vi "cwlaserOnOff.vi"(2 "error in":errorcluster, 3 "Laser On/Off":bool, 4 "cwlaser in":refnum<visa-resource-name>) -> (0 "error out":errorcluster, 1 "cwlaser out":refnum<visa-resource-name>)   [LabVIEW 2017]
panel:
  out "read buffer 3":string
  out "read buffer 2":string
  out "read buffer":string
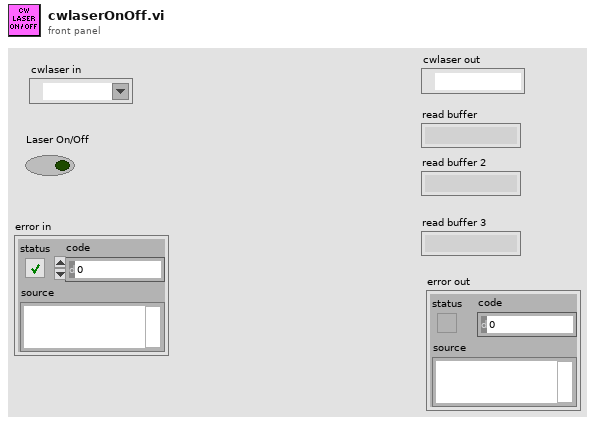
[diagram p1: front panel]
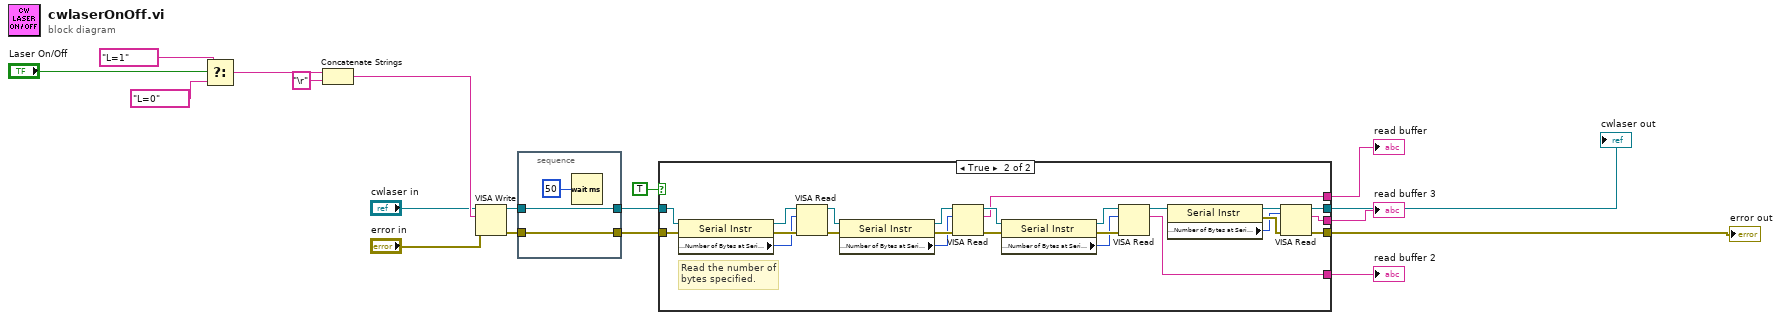
[diagram p0: block diagram]
diagram:
  n1 = Select(t="L=1" ("OutString"), s="Laser On/Off", f="L=0" ("OutString")) -> (s? t:f=w4:string)
  n2 = Concatenate Strings "Concatenate Strings"(w4, "\r") -> (w11:string)
  n3 = VISA Write(VISA resource name="cwlaser in", write buffer=w11, error in (no error)="error in") -> (VISA resource name out=w15:refnum<visa-resource-name>, error out=w14:errorcluster)  [unwired: 1 out]
  n4 = stacked-sequence {
    tunnel: w14 -> [w21]
    tunnel: [w21] -> w16
    tunnel: w15 -> [w20]
    tunnel: [w20] -> w17
    frame #0 {
      n5 = Wait (ms)(milliseconds to wait=u32 50 ("delay before read (ms)")) -> ()  [unwired: 1 out]
    }
  }
  n6 = case shown="True" TRUE ("read") {
    tunnel: w16 -> [w23 w35]
    tunnel: [w23 w25] -> w8
    tunnel: [w22 w26] -> w1
    tunnel: w17 -> [w22 w36]
    tunnel: [_ w37] -> w10
    tunnel: [_ w31] -> w13
    tunnel: [_ w24] -> w12
    frame False {
    }
    frame True {
      # "Read the number of bytes specified."
      n7 = property class="Serial Instr"(reference=w36, error in=w35) -> (reference out=w34:refnum<visa-resource-name>, error out=w33:errorcluster, "Serial Settings:Number of Bytes at Serial Port"=w32:u32)
      n8 = VISA Read(VISA resource name=w34, byte count=w32, error in (no error)=w33) -> (VISA resource name out=w41:refnum<visa-resource-name>, error out=w40:errorcluster)  [unwired: 2 out]
      n9 = property class="Serial Instr"(reference=w41, error in=w40) -> (reference out=w43:refnum<visa-resource-name>, error out=w42:errorcluster, "Serial Settings:Number of Bytes at Serial Port"=w39:u32)
      n10 = VISA Read(VISA resource name=w43, byte count=w39, error in (no error)=w42) -> (VISA resource name out=w45:refnum<visa-resource-name>, read buffer=w37:string, error out=w44:errorcluster)  [unwired: 1 out]
      n11 = property class="Serial Instr"(reference=w45, error in=w44) -> (reference out=w47:refnum<visa-resource-name>, error out=w46:errorcluster, "Serial Settings:Number of Bytes at Serial Port"=w38:u32)
      n12 = VISA Read(VISA resource name=w47, byte count=w38, error in (no error)=w46) -> (VISA resource name out=w27:refnum<visa-resource-name>, read buffer=w31:string)  [unwired: 2 out]
      n13 = property class="Serial Instr"(reference=w27) -> (reference out=w30:refnum<visa-resource-name>, error out=w29:errorcluster, "Serial Settings:Number of Bytes at Serial Port"=w28:u32)  [unwired: 1 in]
      n14 = VISA Read(VISA resource name=w30, byte count=w28, error in (no error)=w29) -> (VISA resource name out=w26:refnum<visa-resource-name>, read buffer=w24:string, error out=w25:errorcluster)  [unwired: 1 out]
    }
  }
  "read buffer" <- w10
  "read buffer 2" <- w13
  "error out" <- w8
  "read buffer 3" <- w12
  "cwlaser out" <- w1
